vi "DSF.Engine.Transfer.Create.vi"(7 "id":i32, 8 "error in (no error)":errorcluster, 9 "String Buffer":refnum<class "DSF.Engine.Memory.Buffer.lvclass">, 10 "Intermediate Buffer":refnum<class "DSF.Engine.Pointer.DBL.lvclass">, 11 "Inline Buffer":refnum<class "DSF.Engine.Pointer.DBL.lvclass">) -> (0 "error out":errorcluster, 3 "Transfer out":refnum<class "DSF.Engine.Transfer.lvclass">)   [LabVIEW 2017, in "DSF.Engine.lvlib" / "DSF.Engine.Transfer.lvclass"]
uses:
  DSF.Engine.Transfer.lvclass
  Buffer/DSF.Engine.Memory.Buffer.lvclass
  Pointer/DSF.Engine.Pointer.DBL.lvclass
  DSF.Engine.Transfer.lvclass/DSF.Engine.Transfer.ctl
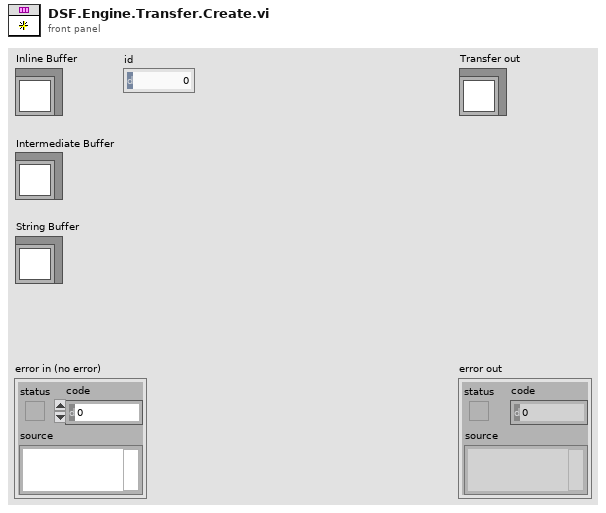
[diagram p1: front panel]
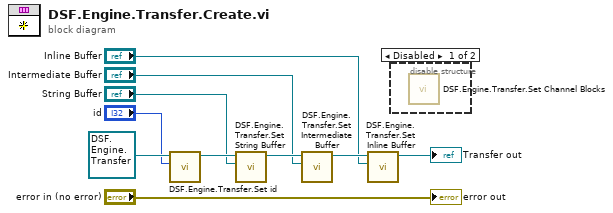
[diagram p0: block diagram]
diagram:
  n1 = call "DSF.Engine.Transfer.Set id.vi"("id"="id", "Transfer in"=refnum<class "DSF.Engine.Transfer.lvclass"> refnum) -> ("Transfer out"=w10:refnum<class "DSF.Engine.Transfer.lvclass">)  [unwired: 9 in]
  n2 = call "DSF.Engine.Transfer.Set String Buffer.vi"("Buffer"="String Buffer", "Transfer in"=w10) -> ("Transfer out"=w8:refnum<class "DSF.Engine.Transfer.lvclass">)  [unwired: 9 in]
  n3 = call "DSF.Engine.Transfer.Set Intermediate Buffer.vi"("DBL Buffer"="Intermediate Buffer", "Transfer in"=w8) -> ("Transfer out"=w7:refnum<class "DSF.Engine.Transfer.lvclass">)  [unwired: 9 in]
  n4 = call "DSF.Engine.Transfer.Set Inline Buffer.vi"("Inline Buffer"="Inline Buffer", "Transfer in"=w7) -> ("Transfer out"=→"Transfer out":refnum<class "DSF.Engine.Transfer.lvclass">)  [unwired: 9 in]
  n5 = disable-structure shown="Disabled" {
    frame Disabled {
      n6 = call "DSF.Engine.Transfer.Set Channel Blocks.vi"() -> ()  [unwired: 11 in, 1 out]
    }
    frame Enabled {
    }
  }
  "error out" <- "error in (no error)"
